vi "CANDLC.vi"(1 "DLC":u8) -> (0 "length":u8)   [LabVIEW 2015]
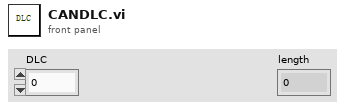
[diagram p1: front panel]
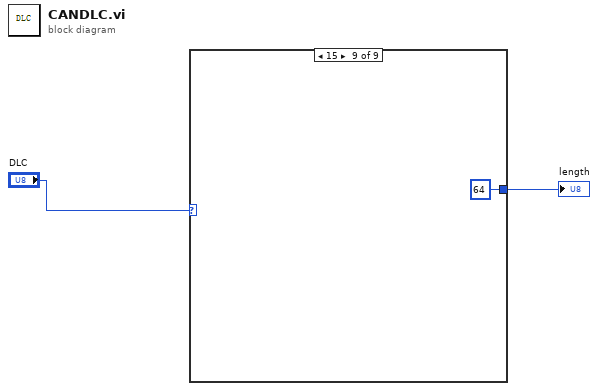
[diagram p0: block diagram]
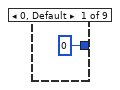
[diagram p2: hidden frame]
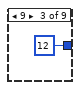
[diagram p4: hidden frame]
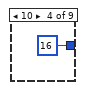
[diagram p5: hidden frame]
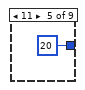
[diagram p6: hidden frame]
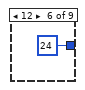
[diagram p7: hidden frame]
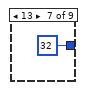
[diagram p8: hidden frame]
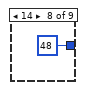
[diagram p9: hidden frame]
diagram:
  n1 = case shown="15" "DLC" {
    selector: "DLC" -> [_ w4 _ _ _ _ _ _ _]
    tunnel: [u8 0 ("DLC") w4 u8 12 ("DLC") u8 16 ("DLC") u8 20 ("DLC") u8 24 ("DLC") u8 32 ("DLC") u8 48 ("DLC") u8 64 ("DLC")] -> w1
    frame 0, Default {
    }
    frame 1..8 {
    }
    frame 9 {
    }
    frame 10 {
    }
    frame 11 {
    }
    frame 12 {
    }
    frame 13 {
    }
    frame 14 {
    }
    frame 15 {
    }
  }
  "length" <- w1
